vi "IDD Test.vi"(5 "aperture time":dbl=0.0167 format="%#_13g", 6 "script name":string="IDD", 7 "SMU Settings":T2={"Level"=1.8, "Level Range"=6.0, "Limit"=0.01, "Limit Range"=0.01, "Sense"=1008} {"Sense" items=["Local"=1008, "Remote"=1009]}, 8 "error in (no error)":errorcluster, 9 "Publishable IDs":string[](array[string])=["IDD_LowPower", "IDD_DVC_Cmin", "IDD_DVC_Cmax"], 10 "Pins":string[](array[string])=["VDD"], 11 "Semiconductor Module Context":T3) -> (0 "error out":errorcluster)   [LabVIEW 2013]
uses:
  <vilib>/NI_TestStand_SemiconductorModule/NI_TestStand_Semiconductor_Module.lvlibp/PinMap/General/SemiconductorModuleContext.ctl
  <instrlib>/niDCPower/nidcpower.llb/niDCPower Sense.ctl
  <instrlib>/niHSDIO/niHSDIO.llb/niHSDIO_ctl Trigger Script - trigID Values (Ring).ctl
  <vilib>/NI_TestStand_SemiconductorModule/NI_TestStand_Semiconductor_Module.lvlibp/PinMap/DC Power/PinsToNIDCPowerSessions.vi
  <vilib>/NI_TestStand_SemiconductorModule/NI_TestStand_Semiconductor_Module.lvlibp/PinMap/General/Publish/PublishDataDouble2D.vi
  <vilib>/NI_TestStand_SemiconductorModule/NI_TestStand_Semiconductor_Module.lvlibp
panel:
  out "current measurements":dbl[][](array[numeric])
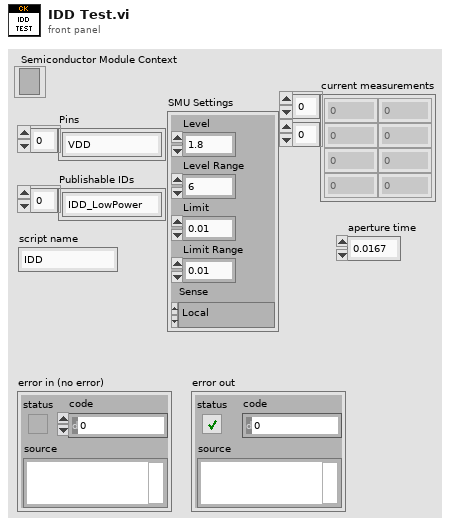
[diagram p1: front panel]
types:
  T1 = typedef "niDCPower Sense.ctl" = i32
  T2 = cluster{"Level":dbl, "Level Range":dbl, "Limit":dbl, "Limit Range":dbl, "Sense":T1}
  T3 = typedef "NI_TestStand_Semiconductor_Module.lvlibp/SemiconductorModuleContext.ctl" = refnum<k7>
  T4 = typedef "niHSDIO_ctl Trigger Script - trigID Values (Ring).ctl" = string
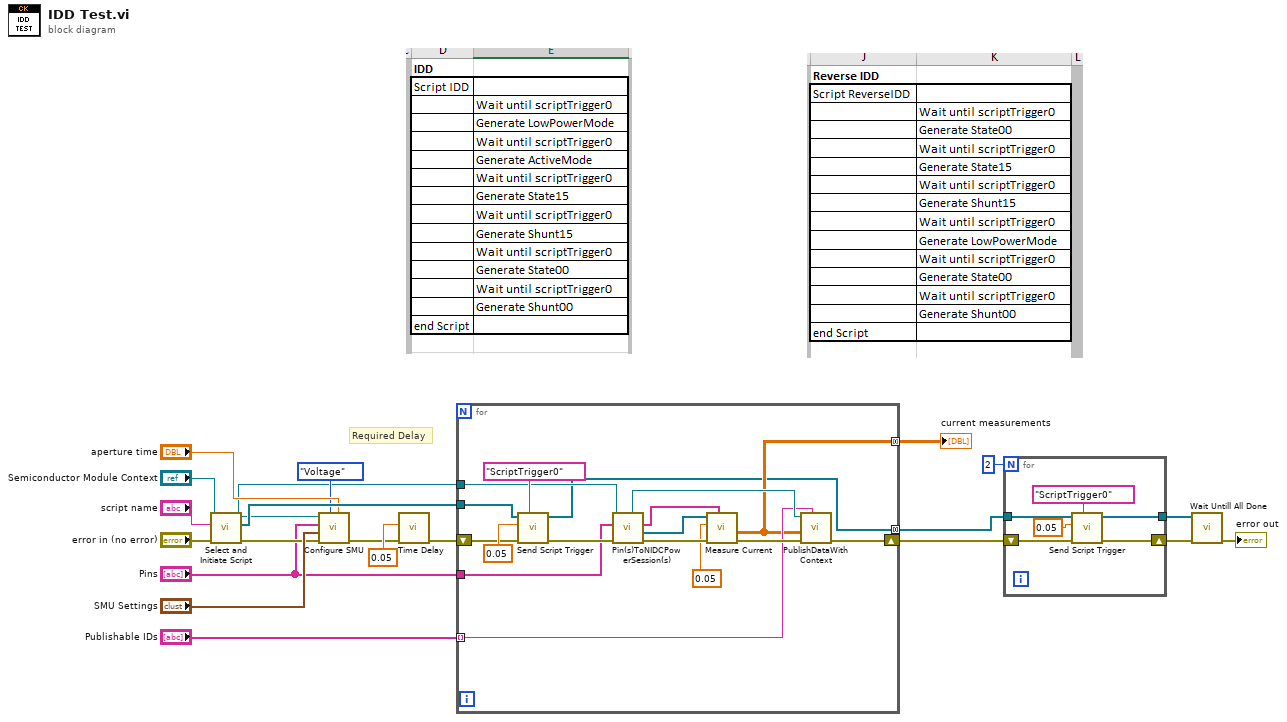
[diagram p0: block diagram]
diagram:
  # "Required Delay"
  n1 = call "Select and Initiate Script.vi"("error in (no error)"="error in (no error)", "script name"="script name", "Semiconductor Module Context"="Semiconductor Module Context") -> ("error out"=w6:errorcluster, "HSDIO GEN Sessions Out"=w16:refnum<k15>[], "Semiconductor Module Context Out"=w2:T3)  [unwired: 6 in]
  n2 = call "Configure SMU.vi"("aperture time"="aperture time", "Source Mode"=enum16{"Voltage", "Current"}."Voltage", "error in (no error)"=w6, "Settings"="SMU Settings", "Pins"="Pins", "Semiconductor Module Context"=w2) -> ("error out"=w4:errorcluster)  [unwired: 5 in]
  n3 = call "Time Delay"("error in (no error)"=w4, "Delay Time (s)"=0.05) -> ("error out"=w3:errorcluster)  [unwired: 9 in]
  n4 = for {
    tunnel: "Pins" -> [w23]
    tunnel: w2 -> [w30]
    tunnel: w16 -> [w22]
    tunnel: "Publishable IDs" -> [w29] mode=indexing
    shift-right: [w33] -> w14
    shift-left: w3 -> [w24]
    tunnel: [w26] -> w17 mode=concatenating
    tunnel: [w25] -> w12 mode=concatenating
    n5 = call "Send Script Trigger.vi"("trigger id (script trigger 0)"=T4 "ScriptTrigger0", "error in (no error)"=w24, "Delay Time (s)"=0.05, "HSDIO Sessions In"=w22) -> ("error out"=w31:errorcluster, "HSDIO Sessions Out"=w25:refnum<k15>[])  [unwired: 6 in]
    n6 = call-poly <vilib>:"Pin(s)ToNIDCPowerSession(s).vi"("error in (no error)"=w31, "Pins"=w23, "Semiconductor Module Context"=w30) -> ("error out"=w34:errorcluster, "Instrument Sessions"=w38:refnum<k15>[], "Channel Lists"=w36:string[], "Pin Query Context"=w35:refnum<class "MultiplePinMultipleSessionQueryContext.lvclass">)  [unwired: 4 in, 1 out]
    n7 = call "Measure Current.vi"("Channel Lists"=w36, "error in (no error)"=w34, "Delay Time (s)"=0.05, "DCPower Sessions In"=w38) -> ("error out"=w37:errorcluster, "current measurements"=w26:dbl[][])  [unwired: 5 in, 1 out]
    n8 = call-poly <vilib>:"PublishDataWithContext.vi"("Published Data Id"=w29, "error in (no error)"=w37, "Data In"=w26, "Pin Query Context"=w35) -> ("error out"=w33:errorcluster)  [unwired: 6 in, 1 out]
  }
  "current measurements" <- w17
  n9 = for {
    N: 2 -> [_]
    tunnel: w12 -> [w42]
    tunnel: [w39] -> w11
    shift-right: [w43] -> w13
    shift-left: w14 -> [w44]
    n10 = call "Send Script Trigger.vi"("trigger id (script trigger 0)"=T4 "ScriptTrigger0", "error in (no error)"=w44, "Delay Time (s)"=0.05, "HSDIO Sessions In"=w42) -> ("error out"=w43:errorcluster, "HSDIO Sessions Out"=w39:refnum<k15>[])  [unwired: 6 in]
  }
  n11 = call "Wait Untill All Done.vi"("error in (no error)"=w13, "HSDIO Sessions In"=w11) -> ("error out"=→"error out":errorcluster)  [unwired: 8 in, 1 out]
